vi "Vision Get Data.vi"() -> ()   [LabVIEW 2016]
uses:
  <vilib>/Rock Robotics/Network Tables/NT Write Number.vi
  <vilib>/Rock Robotics/Network Tables/NT Write String.vi
panel:
  in  "Input Data test":string
  out "Center X 2":dbl
  out "Center Y 2":dbl
  out "Distance 2":dbl
  out "Image In":string
  out "Distance":dbl
  out "Center Y":dbl
  out "Center X":dbl
  out "Data In":string
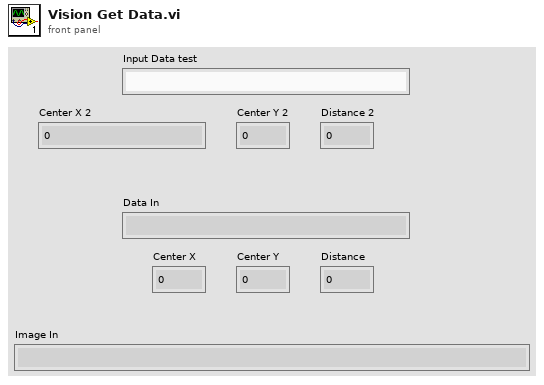
[diagram p1: front panel]
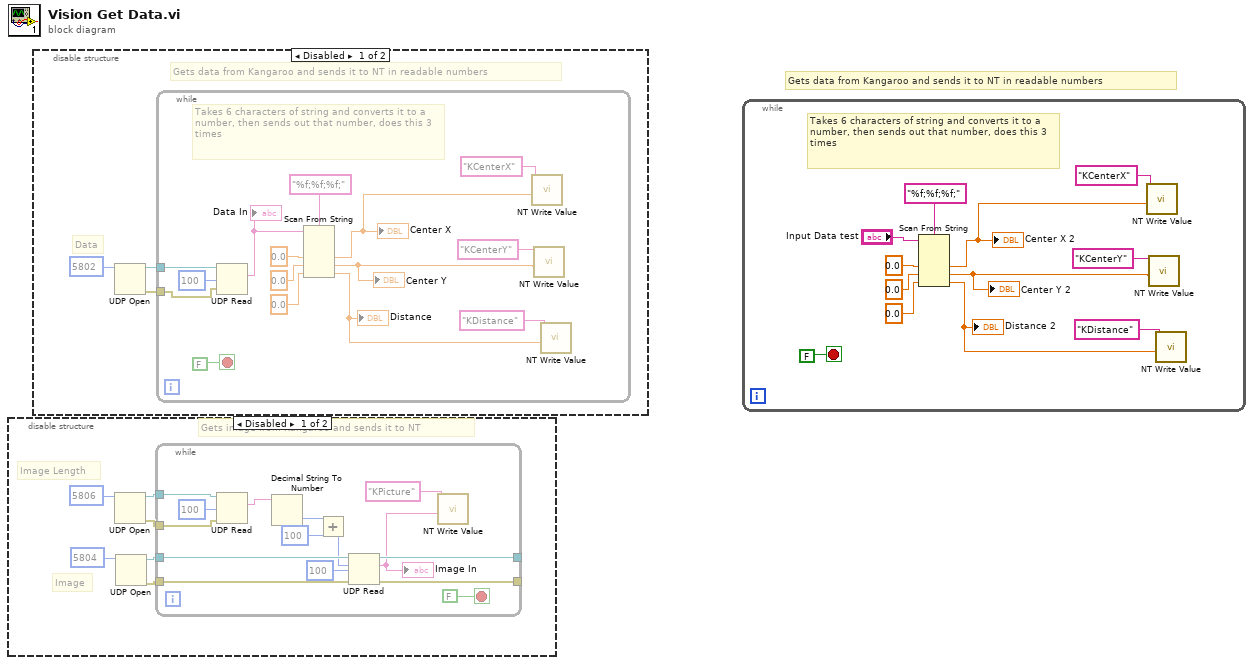
[diagram p0: block diagram]
diagram:
  # "Gets data from Kangaroo and sends it to NT in readable numbers"
  n1 = disable-structure shown="Disabled" {
    frame Disabled {
      # "Image"
      # "Image Length"
      # "Gets image from Kangaroo and sends it to NT"
      n2 = UDP Open(11:u16 5806 ("port")) -> (port=w4:refnum<k16>, 0:w5:errorcluster)  [unwired: 4 in, 1 out]
      n3 = UDP Open(11:u16 5804 ("port")) -> (port=w3:refnum<k16>, 0:w2:errorcluster)  [unwired: 4 in, 1 out]
      n4 = while {
        tunnel: w5 -> [w20]
        tunnel: w4 -> [w19]
        tunnel: w2 -> [w17]
        tunnel: w3 -> [w18]
        tunnel: [w10] -> _
        tunnel: [w9] -> _
        stop <- FALSE stop-if-true
        n5 = UDP Read(connection ID=w19, timeout ms (25000)=100, 8:w20) -> (data out=w15:string)  [unwired: 1 in, 4 out]
        n6 = Decimal String To Number(string=w15) -> (number=w14:i32)  [unwired: 2 in, 1 out]
        n7 = Add(x=w14, y=100) -> (x+y=w12:i32)
        n8 = UDP Read(connection ID=w18, max size (548)=w12, timeout ms (25000)=100, 8:w17) -> (data out=w7:string, error out=w10:errorcluster, 3:w9:refnum<k16>)  [unwired: 2 out]
        "Image In" <- w7
        n9 = call-poly <vilib>:"NT Write Value.vi"("String"=w7, "Name"="KPicture") -> ()  [unwired: 9 in, 1 out]
      }
    }
    frame Enabled {
    }
  }
  n10 = disable-structure shown="Disabled" {
    frame Disabled {
      # "Data"
      # "Gets data from Kangaroo and sends it to NT in readable numbers"
      n11 = UDP Open(11:u16 5802 ("port")) -> (port=w24:refnum<k16>, 0:w23:errorcluster)  [unwired: 4 in, 1 out]
      n12 = while {
        tunnel: w24 -> [w27]
        tunnel: w23 -> [w26]
        stop <- FALSE stop-if-true
        # "Takes 6 characters of string and converts it to a number, then sends out that number, does this 3 times"
        n13 = UDP Read(connection ID=w27, timeout ms (25000)=100, 8:w26) -> (data out=w25:string)  [unwired: 1 in, 4 out]
        "Data In" <- w25
        n14 = Scan From String(format string="%f;%f;%f;", input string=w25, default 1=0.0 ("default value 1"), default 2=0.0 ("default value 2"), default 3=0.0 ("default value 3")) -> (output 1=w29:dbl, output 2=w30:dbl, output 3=w31:dbl)  [unwired: 2 in, 3 out]
        "Center X" <- w29
        "Center Y" <- w30
        "Distance" <- w31
        n15 = call-poly <vilib>:"NT Write Value.vi"("Numeric"=w29, "Name"="KCenterX") -> ()  [unwired: 9 in, 1 out]
        n16 = call-poly <vilib>:"NT Write Value.vi"("Numeric"=w30, "Name"="KCenterY") -> ()  [unwired: 9 in, 1 out]
        n17 = call-poly <vilib>:"NT Write Value.vi"("Numeric"=w31, "Name"="KDistance") -> ()  [unwired: 9 in, 1 out]
      }
    }
    frame Enabled {
    }
  }
  n18 = while {
    stop <- FALSE stop-if-true
    # "Takes 6 characters of string and converts it to a number, then sends out that number, does this 3 times"
    n19 = Scan From String(format string="%f;%f;%f;", input string="Input Data test", default 1=0.0 ("default value 1"), default 2=0.0 ("default value 2"), default 3=0.0 ("default value 3")) -> (output 1=w41:dbl, output 2=w42:dbl, output 3=w43:dbl)  [unwired: 2 in, 3 out]
    "Center X 2" <- w41
    "Center Y 2" <- w42
    "Distance 2" <- w43
    n20 = call-poly <vilib>:"NT Write Value.vi"("Numeric"=w41, "Name"="KCenterX") -> ()  [unwired: 9 in, 1 out]
    n21 = call-poly <vilib>:"NT Write Value.vi"("Numeric"=w42, "Name"="KCenterY") -> ()  [unwired: 9 in, 1 out]
    n22 = call-poly <vilib>:"NT Write Value.vi"("Numeric"=w43, "Name"="KDistance") -> ()  [unwired: 9 in, 1 out]
  }
